vi "Format Error String.vi"(11 "raw error string":string) -> (3 "formatted error string":string)   [LabVIEW 2017, in "Message Log.lvclass"]
uses:
  Message Log.lvclass
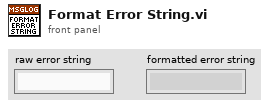
[diagram p1: front panel]
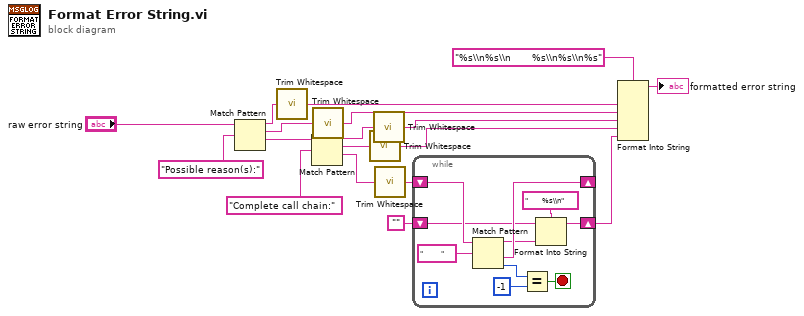
[diagram p0: block diagram]
diagram:
  n1 = Match Pattern(string="raw error string", regular expression="Possible reason(s):") -> (before substring=w16:string, match substring=w10:string, after substring=w8:string)  [unwired: 1 in, 1 out]
  n2 = call <vilib>:"Trim Whitespace.vi"("string"=w16) -> ("trimmed string"=w14:string)  [unwired: 1 in]
  n3 = Match Pattern(string=w8, regular expression="Complete call chain:") -> (before substring=w13:string, match substring=w11:string, after substring=w7:string)  [unwired: 1 in, 1 out]
  n4 = call <vilib>:"Trim Whitespace.vi"("string"=w10) -> ("trimmed string"=w9:string)  [unwired: 1 in]
  n5 = call <vilib>:"Trim Whitespace.vi"("string"=w11) -> ("trimmed string"=w12:string)  [unwired: 1 in]
  n6 = call <vilib>:"Trim Whitespace.vi"("string"=w13) -> ("trimmed string"=w3:string)  [unwired: 1 in]
  n7 = call <vilib>:"Trim Whitespace.vi"("string"=w7) -> ("trimmed string"=w6:string)  [unwired: 1 in]
  n8 = while {
    shift-right: [w24] -> _
    shift-left: w6 -> [w25]
    shift-right: [w20] -> w4
    shift-left: "" -> [w19]
    stop <- w26 stop-if-true
    n9 = Match Pattern(string=w25, regular expression="         ") -> (before substring=w21:string, after substring=w24:string, offset past match=w28:i32)  [unwired: 1 in, 1 out]
    n10 = Equal?(x=w28, y=-1) -> (x = y?=w26:bool)
    n11 = Format Into String(format string="       %s\\n", initial string=w19, w21) -> (resulting string=w20:string)  [unwired: 1 in, 1 out]
  }
  n12 = Format Into String(format string="%s\\n%s\\n       %s\\n%s\\n%s", w14, w9, w3, w12, w4) -> (resulting string=→"formatted error string":string)  [unwired: 2 in, 1 out]
